vi "Generate Tags.vi"(8 "error in (no error)":errorcluster, 10 "Value":i32, 11 "Logger in.lvclass":refnum<class "Logger.lvclass">) -> (0 "error out":errorcluster, 3 "Logger out.lvclass":refnum<class "Logger.lvclass">)   [LabVIEW 2017, in "Logger.lvclass"]
uses:
  Logger.lvclass
  Logger.lvclass/Logger.ctl
  <vilib>/Skyline/Tag/Wrapper/Wrapper_class/Generate Tag Cluster (I32) 2.vi
  <vilib>/Skyline/Tag/Wrapper/Wrapper_class/NI Skyline Tag.lvclass
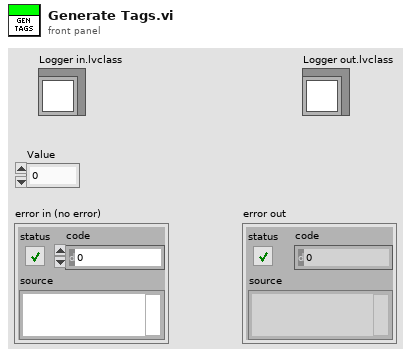
[diagram p1: front panel]
types:
  T1 = typedef "NI Skyline Tag.lvclass/Tag Value Cluster Wrapper.ctl" = cluster{"Configuration":refnum<class "NI Skyline Configuration.lvclass">, "Tag Cluster":T2}
  T2 = typedef "NI Skyline Tag.lvlib/Tag Value Cluster.ctl" = cluster{"Path":string, "Data Type":T3, "Value":string, "Time Stamp":timestamp}
  T3 = typedef "NI Skyline Tag.lvlib/DataType.ctl" = enum32{"Double", "Integer", "String"}
  T4 = cluster{"tag_updates":i32, "tag_publish_interval":i32, "tag_count":i32}
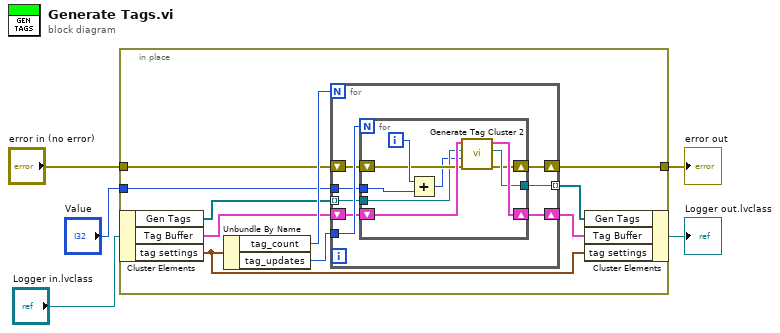
[diagram p0: block diagram]
diagram:
  n1 = in-place {
    in-place-border: "error in (no error)" -> [w12]
    in-place-border: [w11] -> w2
    in-place-border: "Value" -> [w8]
    n2 = in-place-cluster #1("Logger in.lvclass") -> ("Gen Tags"=w7:refnum<class "NI Skyline Tag.lvclass">[], "Tag Buffer"=w10:T1[], "tag settings"=w15:T4)
    n3 = Unbundle By Name(w15) -> ("tag_count"=w14:i32, "tag_updates"=w13:i32)
    n4 = for {
      N: w14 -> [_]
      tunnel: w13 -> [w23]
      shift-right: [w20] -> w11
      shift-left: w12 -> [w17]
      shift-right: [w21] -> w9
      shift-left: w10 -> [w22]
      tunnel: w8 -> [w19]
      tunnel: w7 -> [w18] mode=indexing
      tunnel: [w16] -> w6 mode=indexing
      n5 = for {
        N: w23 -> [_]
        shift-right: [w30] -> w21
        shift-left: w22 -> [w27]
        tunnel: w18 -> [w25]
        shift-right: [w28] -> w20
        shift-left: w17 -> [w26]
        tunnel: w19 -> [w31]
        tunnel: [w29] -> w16
        i -> [w32]
        n6 = Add(x=w32, y=w31) -> (x+y=w24:i32)
        n7 = call-poly <vilib>:"Generate Tag Cluster 2.vi"("error in (no error)"=w26, "value"=w24, "tag in"=w25, "tag clusters in"=w27) -> ("error out"=w28:errorcluster, "tag out"=w29:refnum<class "NI Skyline Tag.lvclass">, "tag clusters out"=w30:T1[])  [unwired: 5 in]
      }
    }
    n8 = in-place-cluster #1("Gen Tags"=w6, "Tag Buffer"=w9, "tag settings"=w15) -> (→"Logger out.lvclass":refnum<class "Logger.lvclass">)
  }
  "error out" <- w2
